vi "Framework Configuration.Initialize.vi"(8 "error in (no error)":errorcluster, 11 "Framework Configuration in":refnum<class "Framework Configuration.lvclass">) -> (0 "error out":errorcluster, 3 "Framework Configuration out":refnum<class "Framework Configuration.lvclass">)   [LabVIEW 2017, in "DSF Core.lvlib" / "Framework Configuration.lvclass"]
uses:
  Framework Configuration.lvclass
  Framework Configuration.lvclass/Framework Configuration.ctl
  Plugin/Plugin Configuration.lvclass
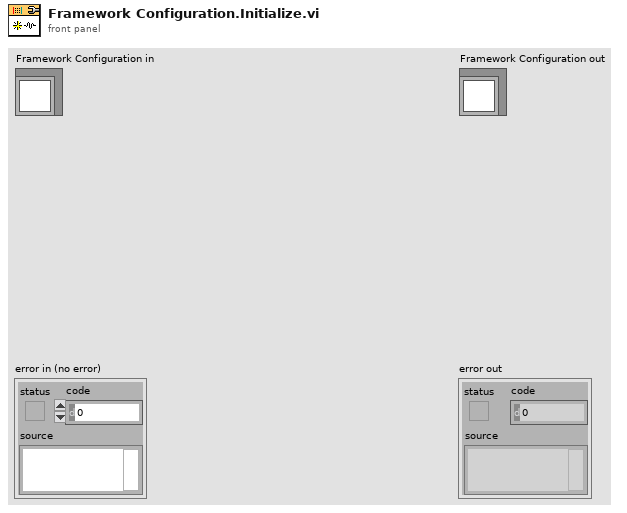
[diagram p1: front panel]
types:
  T1 = typedef "DSF Core.lvlib/DSF Engine Framework Configuration.ctl" = cluster{"Plugins":T2[]}
  T2 = typedef "DSF Core.lvlib/DSF Engine Plugin Configuration.ctl" = cluster{"name":string, "class":string, "cycle timing":T3, "Transfer Groups":T4[], "settings":T10}
  T3 = typedef "DSF Core.lvlib/DSF Timing Info.ctl" = cluster{"priority":u64, "decimation":u64, "offset":u64}
  T4 = typedef "DSF Core.lvlib/DSF Engine Transfer Group Configuration.ctl" = cluster{"name":string, "direction":T5, "cycle timing":T3, "Transfers":T6[], "settings":T10}
  T5 = typedef "DSF Core.lvlib/DSF Direction.ctl" = enum8{"Tx", "Rx"}
  T6 = typedef "DSF Core.lvlib/DSF Engine Transfer Configuration.ctl" = cluster{"name":string, "byte order":T7, "channel configurations":T8[], "settings":T10}
  T7 = typedef "DSF Core.lvlib/DSF Byte Order.ctl" = enum8{"big-endian", "little-endian"}
  T8 = typedef "DSF Core.lvlib/DSF Engine Channel Configuration.ctl" = cluster{"engine offset":u64, "name":string, "data type":T9, "count":u64, "buffer offset":u64, "settings":T10}
  T9 = typedef "DSF Core.lvlib/DSF Data Type.ctl" = enum8{"Bool", "SGL", "DBL", "I8", "I16", "I32", "I64", "U8", "U16", "U32", "U64"}
  T10 = typedef "DSF Core.lvlib/DSF Settings Info.ctl" = cluster{"key":string, "value":string}[]
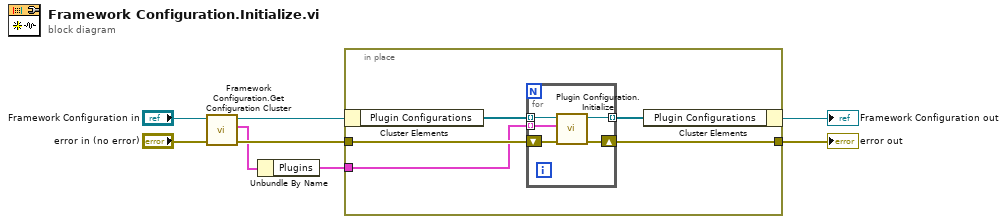
[diagram p0: block diagram]
diagram:
  n1 = call "Framework Configuration.Get Configuration Cluster.vi"("Framework Configuration in"="Framework Configuration in") -> ("Framework Configuration"=w2:T1, "Framework Configuration out"=w3:refnum<class "Framework Configuration.lvclass">)  [unwired: 9 in]
  n2 = Unbundle By Name(w2) -> ("Plugins"=w1:T2[])
  n3 = in-place {
    in-place-border: "error in (no error)" -> [w10]
    in-place-border: [w9] -> w6
    in-place-border: w1 -> [w8]
    n4 = in-place-cluster #1(w3) -> ("Plugin Configurations"=w12:refnum<class "Plugin Configuration.lvclass">[])
    n5 = for {
      tunnel: w12 -> [w17] mode=indexing
      tunnel: [w16] -> w11 mode=indexing
      shift-right: [w15] -> w9
      shift-left: w10 -> [w14]
      tunnel: w8 -> [w13] mode=indexing
      n6 = call-dynamic "Plugin Configuration.Initialize.vi"("error in (no error)"=w14, "Plugin Configuration cluster"=w13, "Plugin Configuration in"=w17) -> ("error out"=w15:errorcluster, "Plugin Configuration"=w16:refnum<class "Plugin Configuration.lvclass">)  [unwired: 7 in]
    }
    n7 = in-place-cluster #1("Plugin Configurations"=w11) -> (→"Framework Configuration out":refnum<class "Framework Configuration.lvclass">)
  }
  "error out" <- w6
